vi "SIM BuildSimErr.vi"(1 "error.code":i32=42, 2 "Additional Details":string, 3 "Block Name":string, 4 "CallChain":string) -> (0 "Error Cluster":errorcluster)   [LabVIEW 2020]
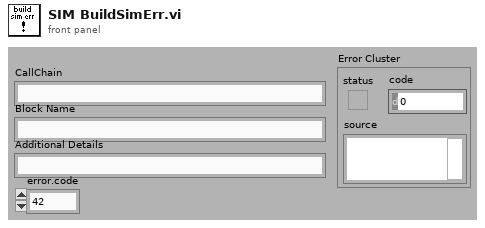
[diagram p1: front panel]
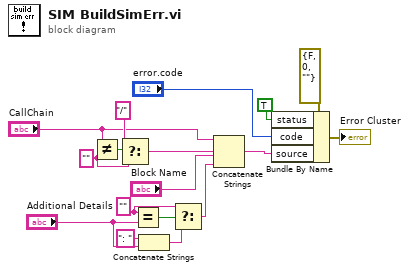
[diagram p0: block diagram]
diagram:
  w4 = "" ("y")
  w11 = "" ("y")
  n1 = Not Equal?(x="CallChain", y=w4) -> (x != y?=w2:bool)
  n2 = Select(t="/" ("string"), s=w2, f=w4) -> (s? t:f=w3:string)
  n3 = Equal?(x=w11, y="Additional Details") -> (x = y?=w12:bool)
  n4 = Concatenate Strings(": " ("string"), "Additional Details") -> (w8:string)
  n5 = Select(t=w11, s=w12, f=w8) -> (s? t:f=w7:string)
  n6 = Concatenate Strings("CallChain", w3, "Block Name", w7) -> (w16:string)
  n7 = Bundle By Name(cluster=errorcluster {"status"=FALSE, "code"=0, "source"=""} ("error"), "status"=TRUE ("error.status"), "code"="error.code", "source"=w16) -> (→"Error Cluster":errorcluster)
